vi "Uninit App.vi"(8 "error in (no error)":errorcluster, 11 "VolatusCore in":refnum<class "VolatusCore.lvclass">) -> (0 "error out":errorcluster, 3 "VolatusCore out":refnum<class "VolatusCore.lvclass">)   [LabVIEW 2020, in "Volatus.lvlib" / "VolatusCore.lvclass"]
uses:
  VolatusCore.lvclass
  VolatusCore.lvclass/VolatusCore.ctl
  App/App.lvclass
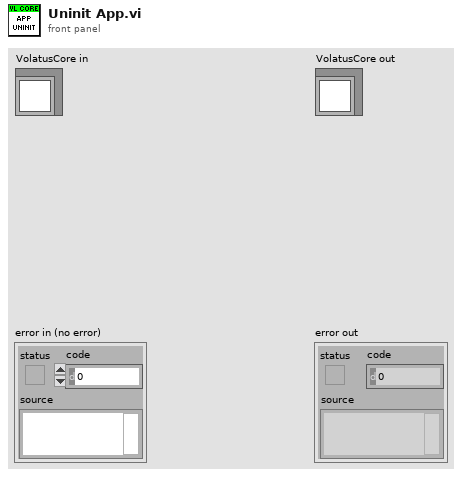
[diagram p1: front panel]
types:
  T1 = typedef "Volatus.lvlib/Core APIs.ctl" = cluster{"Volatus":refnum<class "VolatusAPI.lvclass">, "Event":refnum<class "EventAPI.lvclass">, "Config":refnum<class "ConfigAPI.lvclass">}
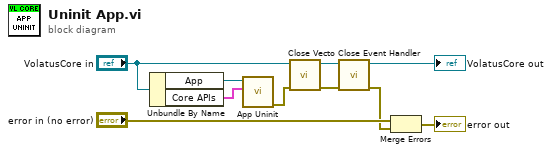
[diagram p0: block diagram]
diagram:
  n1 = Unbundle By Name("VolatusCore in") -> ("App"=w10:refnum<class "App.lvclass">, "Core APIs"=w9:T1)
  n2 = call-dynamic "App Uninit.vi"("Core APIs"=w9, "App in"=w10) -> ("error out"=w2:errorcluster)  [unwired: 9 in]
  n3 = call "Close Vecto.vi"("error in (no error)"=w2, "VolatusCore in"="VolatusCore in") -> ("error out"=w6:errorcluster, "VolatusCore out"=w5:refnum<class "VolatusCore.lvclass">)  [unwired: 8 in]
  n4 = call "Close Event Handler.vi"("error in (no error)"=w6, "VolatusCore in"=w5) -> ("error out"=w1:errorcluster, "VolatusCore out"=→"VolatusCore out":refnum<class "VolatusCore.lvclass">)  [unwired: 8 in]
  n5 = Merge Errors("error in (no error)", w1) -> (→"error out":errorcluster)
